vi "ArraytoIgorWave.vi"   [LabVIEW 2019]
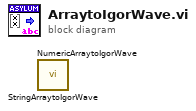
[diagram p0: block diagram]
diagram:
  n1 = call "StringArraytoIgorWave.vi"() -> ()  [unwired: 10 in, 2 out]
  n2 = call "NumericArraytoIgorWave.vi"() -> ()  [unwired: 10 in, 2 out]
